vi "Create simplified GUI element.vi"(8 "error in (no error)":errorcluster, 10 "Index":i32, 11 "Scan SBlock in":refnum<class "Scan SBlock.lvclass">) -> (0 "error out":errorcluster, 2 "Simple GUI Element":T1={"Bcg Color"=16777225, "Index"=0, "No. of runs"=0, "Script name"="", "FPGA name"="", "Parameters"="", "Repetitions"=0}, 3 "Scan SBlock out":refnum<class "Scan SBlock.lvclass">)   [LabVIEW 2020, in "Run Utilities.lvlib" / "Scan SBlock.lvclass"]
doc: "Create a GUI element for this SBlock"
uses:
  Scan SBlock.lvclass
  Schedule Block/Schedule Block.lvclass
  Scan SBlock.lvclass/Scan SBlock.ctl
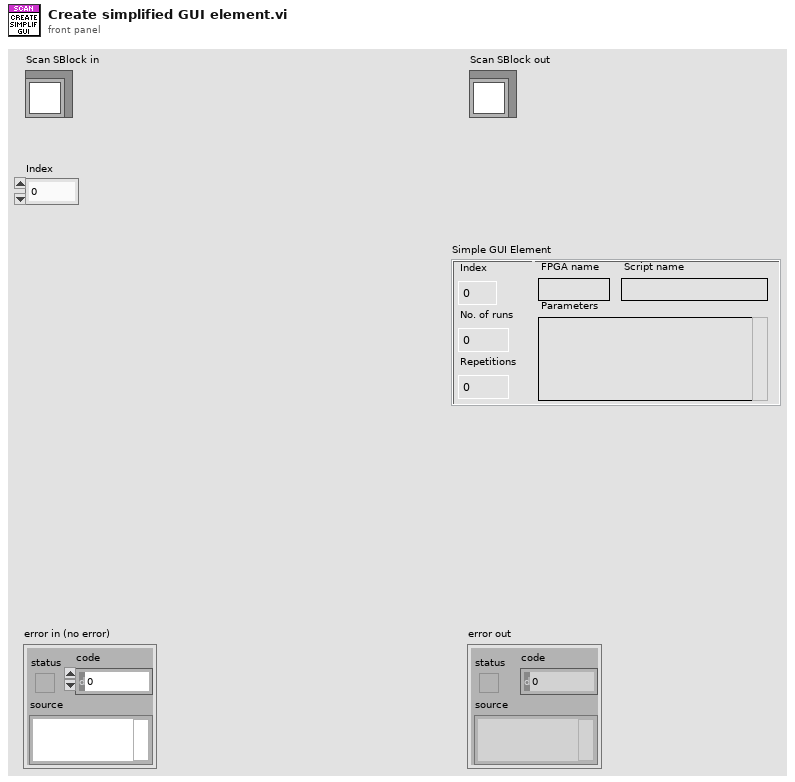
[diagram p1: front panel]
types:
  T1 = cluster{"Bcg Color":u32, "Index":i32, "No. of runs":i32, "Script name":string, "FPGA name":string, "Parameters":string, "Repetitions":i32}
  T2 = typedef "Run Utilities.lvlib/Schedule Block.lvclass/Schedule Block - simplified GUI.ctl" = cluster{"Bcg Color":u32, "Index":i32, "No. of runs":i32, "Script name":string, "FPGA name":string, "Parameters":string, "Repetitions":i32}
  T3 = typedef "Run Utilities.lvlib/Scan SBlock.lvclass/Advanced Parameters.ctl" = cluster{"Param":string, "From":dbl, "To":dbl, "Step":dbl, "Mode":T4}
  T4 = typedef "Run Utilities.lvlib/Scan SBlock.lvclass/Advanced Panel Parameter Mode.ctl" = enum16{"Linear", "Log", "LINKED"}
  T5 = typedef "Run Utilities.lvlib/Scan SBlock.lvclass/Advanced Parameters - list.ctl" = cluster{"Param":string, "List of values":string[]}
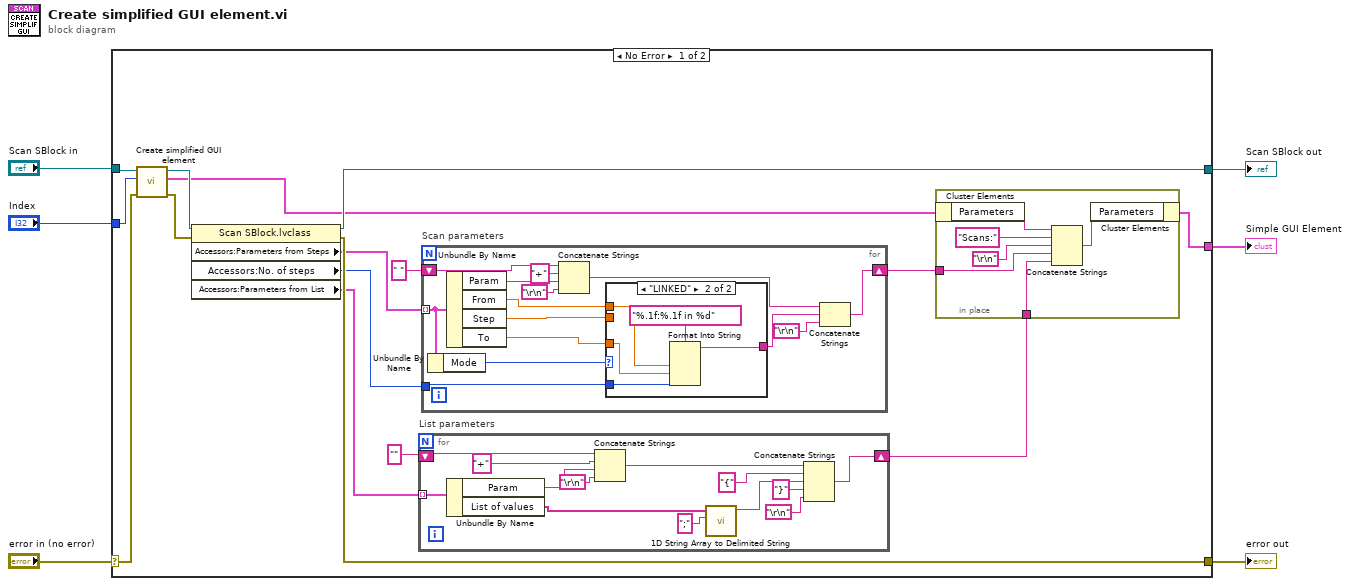
[diagram p0: block diagram]
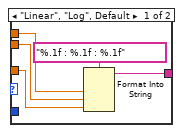
[diagram p2: hidden frame]
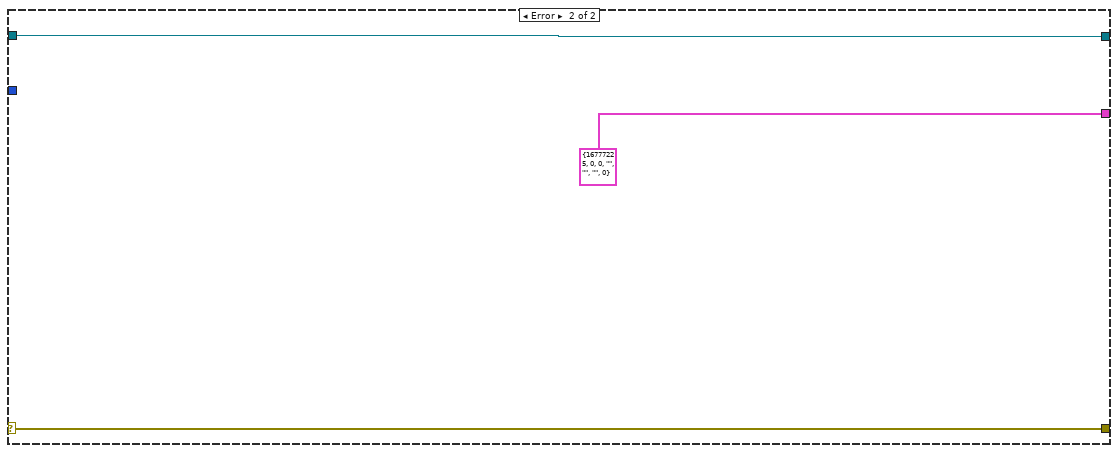
[diagram p3: hidden frame]
diagram:
  n1 = case shown="No Error" "error in (no error)" {
    selector: "error in (no error)" -> [w11 w68]
    tunnel: [w21 w68] -> w3
    tunnel: [w22 w67] -> w5
    tunnel: "Scan SBlock in" -> [w13 w67]
    tunnel: [w7 T1 {"Bcg Color"=16777225, "Index"=0, "No. of runs"=0, "Script name"="", "FPGA name"="", "Parameters"="", "Repetitions"=0} ("Cluster")] -> w4
    tunnel: "Index" -> [w12 _]
    frame No Error {
      n2 = call-parent "Create simplified GUI element.vi"("error in (no error)"=w11, "Index"=w12, "Schedule Block in"=w13) -> ("error out"=w10:errorcluster, "Simple GUI Element"=w8:T2, "Schedule Block out"=w9:refnum<class "Scan SBlock.lvclass">)  [unwired: 6 in]
      n3 = property class="Scan SBlock.lvclass"(reference=w9, error in=w10) -> (reference out=w22:refnum<class "Scan SBlock.lvclass">, error out=w21:errorcluster, "Accessors:Parameters from Steps"=w14:T3[], "Accessors:No. of steps"=w16:u32, "Accessors:Parameters from List"=w15:T5[])
      n4 = for "List parameters" {
        tunnel: w15 -> [w41] mode=indexing
        shift-right: [w37] -> w17
        shift-left: "" -> [w36]
        n5 = Unbundle By Name(w41) -> ("Param"=w40:string, "List of values"=w34:string[])
        n6 = Concatenate Strings(w36, "+" ("string"), w40, "\r\n") -> (w38:string)
        n7 = call <vilib>:"1D String Array to Delimited String.vi"("delimiter"=";", "string array"=w34) -> ("delimited string"=w32:string)  [unwired: 9 in]
        n8 = Concatenate Strings(w38, "{" ("string"), w32, "}" ("string"), "\r\n") -> (w37:string)
      }
      n9 = for "Scan parameters" {
        tunnel: w14 -> [w54] mode=indexing
        shift-right: [w45] -> w19
        shift-left: " " -> [w43]
        tunnel: w16 -> [w44]
        n10 = Unbundle By Name(w54) -> ("Mode"=w55:T4)
        n11 = Unbundle By Name(w54) -> ("Param"=w53:string, "From"=w51:dbl, "Step"=w50:dbl, "To"=w49:dbl)
        n12 = Concatenate Strings(w43, "+" ("string"), w53, "\r\n") -> (w47:string)
        n13 = case shown="\"LINKED\"" w55 {
          tunnel: w51 -> [w60 w64]
          tunnel: w50 -> [w58 _]
          tunnel: w49 -> [w57 w65]
          tunnel: [w56 w62] -> w46
          tunnel: w44 -> [_ w61]
          frame "Linear", "Log", Default {
            n14 = Format Into String(format string="%.1f : %.1f : %.1f", w60, w58, w57) -> (resulting string=w56:string)  [unwired: 2 in, 1 out]
          }
          frame "LINKED" {
            n15 = Format Into String(format string="%.1f:%.1f in %d", w64, w65, w61) -> (resulting string=w62:string)  [unwired: 2 in, 1 out]
          }
        }
        n16 = Concatenate Strings(w47, w46, "\r\n") -> (w45:string)
      }
      n17 = in-place {
        in-place-border: w19 -> [w26]
        in-place-border: w17 -> [w25]
        n18 = in-place-cluster #1(w8) -> ("Parameters"=w24:string)
        n19 = Concatenate Strings(w24, "Scans:" ("string"), "\r\n", w26, w25) -> (w23:string)
        n20 = in-place-cluster #1("Parameters"=w23) -> (w7:T2)
      }
    }
    frame Error {
    }
  }
  "error out" <- w3
  "Scan SBlock out" <- w5
  "Simple GUI Element" <- w4
